vi "insert_preamble.vi"(8 "error in (no error)":errorcluster, 10 "Payload":i8[](array[numeric]) caption="Key Bit Sequence", 11 "Modulation Parameters In":T1) -> (0 "error out":errorcluster, 1 "Preamble":i8[](array[numeric]), 2 "Transmitted Bit Sequence":i8[](array[numeric]), 3 "Modulation Parameters  Out":T1)   [LabVIEW 2012]
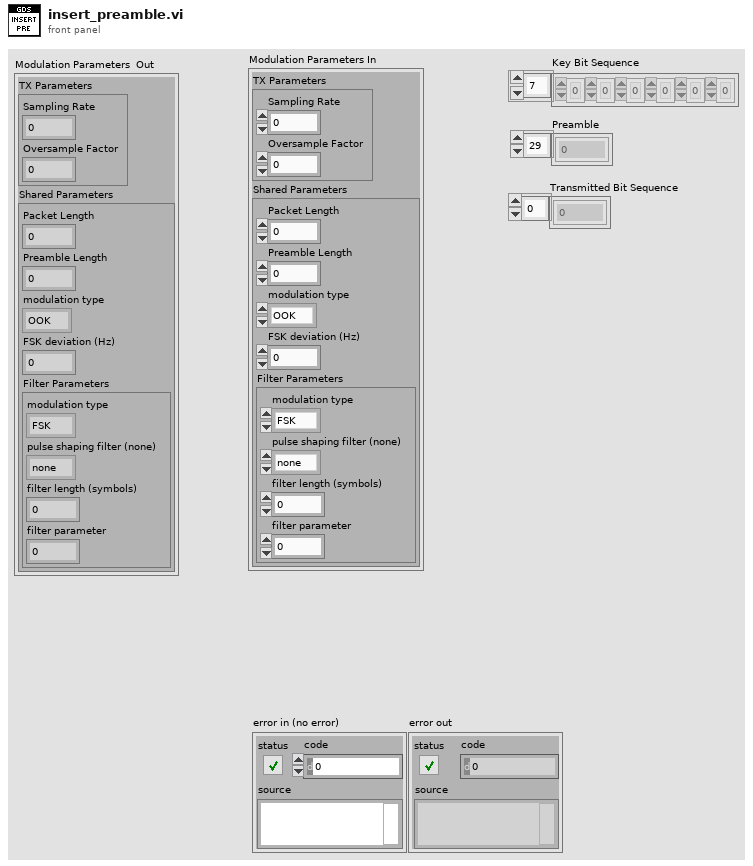
[diagram p1: front panel]
types:
  T1 = cluster{"TX Parameters":cluster{"Sampling Rate":dbl, "Oversample Factor":i32}, "Shared Parameters":cluster{"Packet Length":i32, "Preamble Length":i32, "modulation type":enum16{"OOK", "FSK", "PSK", "QAM", "MSK", "PAM", "ASK", "CPM"}, "FSK deviation (Hz)":dbl, "Filter Parameters":cluster{"modulation type":enum16{"FSK", "PSK", "QAM", "MSK", "PAM", "ASK", "CPM"}, "pulse shaping filter (none)":enum16{"none", "Raised Cosine", "Root Raised Cos", "Gaussian"}, "filter length (symbols)":i32, "filter parameter":dbl}}}
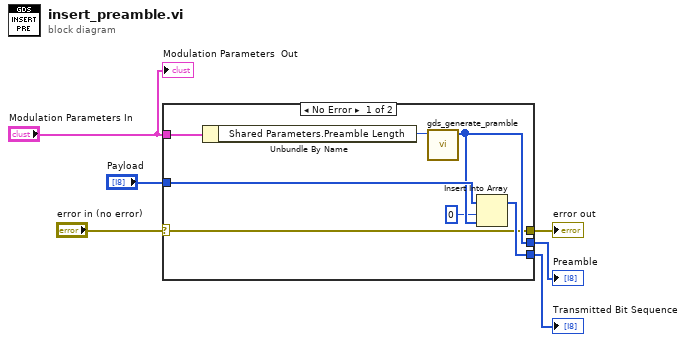
[diagram p0: block diagram]
diagram:
  n1 = case shown="No Error" "error in (no error)" {
    selector: "error in (no error)" -> [w7 w14]
    tunnel: [w7 w14] -> w5
    tunnel: "Modulation Parameters In" -> [w13 _]
    tunnel: [w9 _] -> w4
    tunnel: [w11 _] -> w3
    tunnel: "Payload" -> [w10 _]
    frame No Error {
      n2 = Unbundle By Name(w13) -> ("Shared Parameters.Preamble Length"=w12:i32)
      n3 = call "gds_generate_pramble.vi"("Preamble Length (bits)"=w12) -> ("Preamble"=w9:i32[])  [unwired: 10 in]
      n4 = Insert Into Array(array=w10, index=0, new element=w9) -> (w11:i8[])
    }
    frame Error {
    }
  }
  "Preamble" <- w4
  "Transmitted Bit Sequence" <- w3
  "error out" <- w5
  "Modulation Parameters  Out" <- "Modulation Parameters In"
